vi "PXI-Channel Index to Physical Channel.vi"(10 "index":i32) -> (2 "element":tag)   [LabVIEW 2020]
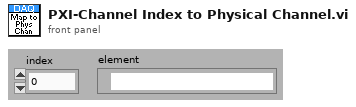
[diagram p1: front panel]
types:
  T1 = cluster{"DAQChan to PhysDev":i32[][], "PhysDev to DAQChan":i32[][]}
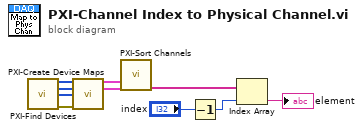
[diagram p0: block diagram]
diagram:
  n1 = call "PXI-Find Devices.vi"() -> ("Num AO"=w8:i32[], "Num AI"=w7:i32[], "Slot Num"=w10:u32[], "error out"=w9:errorcluster)  [unwired: 12 in]
  n2 = call "PXI-Create Device Maps.vi"("Num AO"=w8, "Num AI"=w7, "Slot Num"=w10, "error in (no error)"=w9) -> ("AO Map"=w5:T1, "AI Map"=w4:T1)  [unwired: 9 in, 1 out]
  n3 = call "PXI-Sort Channels.vi"("AO Map"=w5, "AI Map"=w4) -> ("Sorted physical channels"=w3:tag[])  [unwired: 12 in, 1 out]
  n4 = Decrement(x="index") -> (x-1=w1:i32)
  n5 = Index Array(array=w3, index=w1) -> (element=→"element":tag)
